vi "Dispose.vi"(8 "Error In":errorcluster, 11 "reference in":refnum<class "BreakfastMenuEnum.lvclass">) -> (0 "Error Out":errorcluster, 3 "reference out":refnum<class "BreakfastMenuEnum.lvclass">)   [LabVIEW 2020, in "BreakfastMenuEnum.lvclass"]
uses:
  BreakfastMenuEnum.lvclass
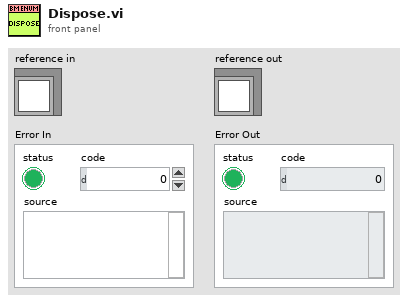
[diagram p1: front panel]
types:
  T1 = typedef "BreakfastMenuEnum.lvclass/ObjectAttributes.ctl" = cluster{"_items":variant[], "_position":i32, "IEnumerator.Current":refnum<class>, "Current":refnum<class "Menu.lvclass">}
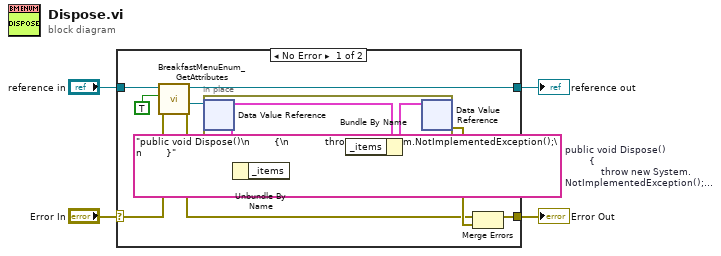
[diagram p0: block diagram]
diagram:
  (unwired) "public void Dispose()\n        {\n            throw new System.NotImplementedException();\n        }"  # public void Dispose()         {             throw new System.NotImplementedException();         }
  n1 = case shown="No Error" "Error In" {
    selector: "Error In" -> [w11 w16]
    tunnel: [w8 w16] -> w3
    tunnel: [w9 w15] -> w1
    tunnel: "reference in" -> [w12 w15]
    frame No Error {
      n2 = call "BreakfastMenuEnum_GetAttributes.vi"("error in (no error)"=w11, "OnlyGetDvrReference(False)"=TRUE, "reference in"=w12) -> ("error out"=w6:errorcluster, "DataRef"=w7:refnum<data-value>, "reference out"=w9:refnum<class "BreakfastMenuEnum.lvclass">)  [unwired: 5 in, 1 out]
      n3 = in-place {
        n4 = in-place-dvr #1(w7) -> (w13:T1)  [unwired: 1 out]
        n5 = Unbundle By Name(w13) -> ()  [unwired: 1 out]
        n6 = Bundle By Name(cluster=w13) -> (w14:T1)  [unwired: 1 in]
        n7 = in-place-dvr #1(w14) -> (w10:errorcluster)  [unwired: 1 out]
      }
      n8 = Merge Errors(w6, w10) -> (w8:errorcluster)
    }
    frame Error {
    }
  }
  "Error Out" <- w3
  "reference out" <- w1
